vi "Initialize EtherCAT youBot Gripper Motor.vi"(7 "index":i32, 8 "error in (no error)":errorcluster, 10 "gripper motor param":T1={"ticks per meter"=1.0, "ticks offset"=0, "StallGuard2Threshold"=50.0, "StallGuard2FilterEnable"=FALSE, "do calibration?"=FALSE, "positive calibtration direction?"=FALSE, "calibration max current (A)"=1.0}, 11 "motor slave info in":T2 {"nodeAddr" format="%.0x"}) -> (0 "error out":errorcluster, 3 "KUKA youBot gripper motor_EtherCAT out":refnum<class "NI_Robotics_KUKA youBot Gripper Motor_EtherCAT.lvclass">)   [LabVIEW 2017, in "NI_Robotics_KUKA youBot Host.lvlib" / "NI_Robotics_KUKA youBot Gripper Motor_EtherCAT.lvclass"]
uses:
  <vilib>/robotics/KUKA youBot/Motor/Gripper Motor EtherCAT/NI_Robotics_KUKA youBot Gripper Motor_EtherCAT.lvclass
  <vilib>/robotics/KUKA youBot/EtherCAT/Motor Slave Info.ctl
  <vilib>/robotics/KUKA youBot/EtherCAT/LowLevel/Mater Handler.ctl
  <vilib>/robotics/KUKA youBot/Motor/Gripper Motor EtherCAT/Gripper Motor Param.ctl
  <vilib>/robotics/KUKA youBot/Motor/Gripper Motor EtherCAT/NI_Robotics_KUKA youBot Gripper Motor_EtherCAT.lvclass/NI_Robotics_KUKA youBot Gripper Motor_EtherCAT.ctl
  <vilib>/robotics/KUKA youBot/NI_Robotics_KUKA youBot Host.lvlib
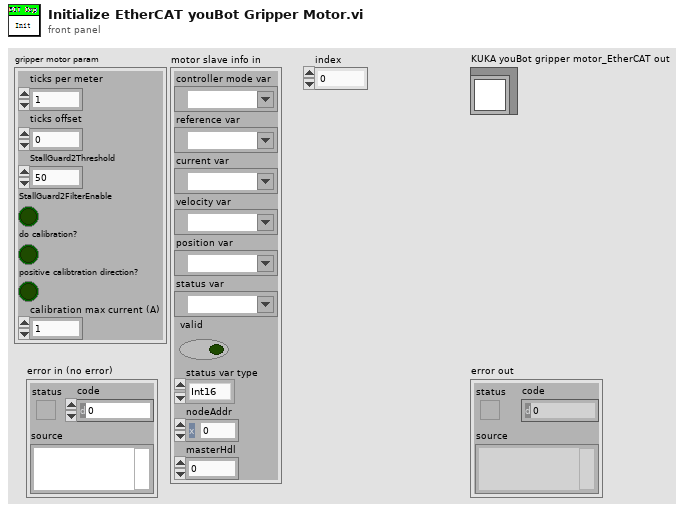
[diagram p1: front panel]
types:
  T1 = typedef "NI_Robotics_KUKA youBot Host.lvlib/NI_Robotics_KUKA youBot Gripper Motor_EtherCAT.lvclass/Gripper Motor Param.ctl" = cluster{"ticks per meter":dbl, "ticks offset":i32, "StallGuard2Threshold":dbl, "StallGuard2FilterEnable":bool, "do calibration?":bool, "positive calibtration direction?":bool, "calibration max current (A)":dbl}
  T2 = typedef "NI_Robotics_KUKA youBot Host.lvlib/Motor Slave Info.ctl" = cluster{"controller mode var":refnum<k21>, "reference var":refnum<k21>, "current var":refnum<k21>, "velocity var":refnum<k21>, "position var":refnum<k21>, "status var":refnum<k21>, "valid":bool, "status var type":enum16{"Int16", "Int32"}, "nodeAddr":u16, "masterHdl":T3}
  T3 = typedef "NI_Robotics_KUKA youBot Host.lvlib/Mater Handler.ctl" = i32
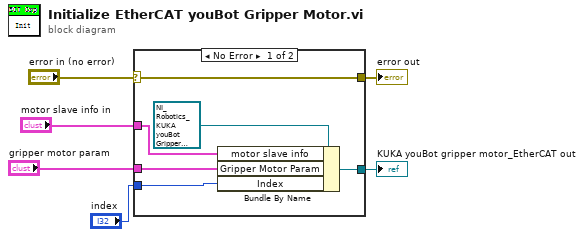
[diagram p0: block diagram]
diagram:
  n1 = case shown="No Error" "error in (no error)" {
    selector: "error in (no error)" -> [w12 w13]
    tunnel: [w12 w13] -> w5
    tunnel: "motor slave info in" -> [w7 _]
    tunnel: "gripper motor param" -> [w10 _]
    tunnel: [w9 _] -> w2
    tunnel: "index" -> [w8 _]
    frame No Error {
      n2 = Bundle By Name(cluster=refnum<class "NI_Robotics_KUKA youBot Gripper Motor_EtherCAT.lvclass"> refnum ("NI_Robotics_KUKA youBot Host.lvlib:NI_Robotics_KUKA youBot Gripper Motor_EtherCAT.lvclass"), "motor slave info"=w7, "Gripper Motor Param"=w10, "Index"=w8) -> (w9:refnum<class "NI_Robotics_KUKA youBot Gripper Motor_EtherCAT.lvclass">)
    }
    frame Error {
    }
  }
  "error out" <- w5
  "KUKA youBot gripper motor_EtherCAT out" <- w2
